vi "Extended Register Read.vi"(0 "instrument handle in":refnum<k15>, 1 "Bus Number":i32, 5 "Slave Address":T3=12 format="%02x", 7 "Register Address":T2 format="%02x", 9 "Byte Count":i32=1, 11 "error in (no error)":errorcluster) -> (4 "instrument handle out":refnum<k15>, 6 "Register Data":T1[](array[typedef]) format="%02x", 15 "error out":errorcluster)   [LabVIEW 2018, in "MIPI RFFE API.lvlib"]
uses:
  Slave Address.ctl
  Register Address.ctl
  Register Data.ctl
  Extended Command/RFFE Extended Command.lvclass/RFFE Extended Command.ctl
  Extended Command/Get Register Data.vi
  RegReadExt/RFFE RegReadExt Command.lvclass
  C:/Users/semoore/Projects/mipi-rffe-labview-oop/Extended Command/RFFE Extended Command.lvclass
  MIPI RFFE API.lvlib
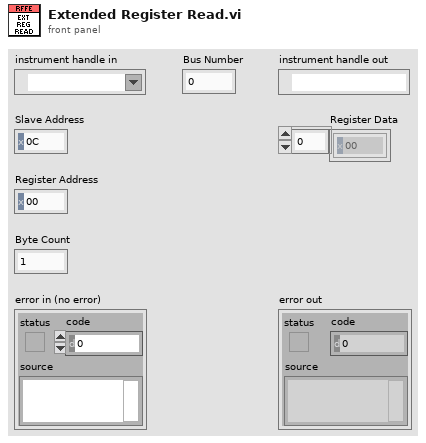
[diagram p1: front panel]
types:
  T1 = typedef "MIPI RFFE API.lvlib/Register Data.ctl" = u8
  T2 = typedef "MIPI RFFE API.lvlib/Register Address.ctl" = u16
  T3 = typedef "MIPI RFFE API.lvlib/Slave Address.ctl" = u8
  T4 = typedef "RFFE Commands.lvlib/Register Data.ctl" = u8
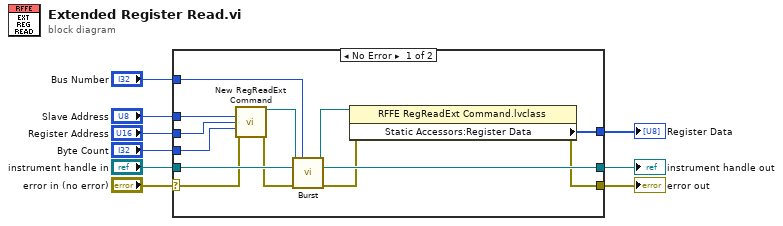
[diagram p0: block diagram]
diagram:
  n1 = case shown="No Error" "error in (no error)" {
    selector: "error in (no error)" -> [w20 w23]
    tunnel: "instrument handle in" -> [w22 w24]
    tunnel: [w21 w24] -> w8
    tunnel: "Slave Address" -> [w18 _]
    tunnel: "Register Address" -> [w17 _]
    tunnel: [w13 w23] -> w4
    tunnel: [w12 _] -> w3
    tunnel: "Byte Count" -> [w11 _]
    tunnel: "Bus Number" -> [w10 _]
    frame No Error {
      n2 = call "New RegReadExt Command.vi"("Slave Address"=w18, "Register Address"=w17, "Byte Count"=w11, "error in (no error)"=w20) -> ("RFFE RegReadExt Command out"=w16:refnum<class "RFFE RegReadExt Command.lvclass">, "error out"=w19:errorcluster)  [unwired: 10 in]
      n3 = call-dynamic "Burst.vi"("RFFE RegReadExt Command in"=w16, "Bus Number"=w10, "instrument handle in"=w22, "error in (no error)"=w19) -> ("RFFE RegReadExt Command out"=w15:refnum<class "RFFE RegReadExt Command.lvclass">, "instrument handle out"=w21:refnum<k15>, "error out"=w14:errorcluster)  [unwired: 9 in]
      n4 = property class="RFFE RegReadExt Command.lvclass"(reference=w15, error in=w14) -> (error out=w13:errorcluster, "Static Accessors:Register Data"=w12:T4[])  [unwired: 1 out]
    }
    frame Error {
    }
  }
  "instrument handle out" <- w8
  "error out" <- w4
  "Register Data" <- w3
